vi "DP-Plot DPGram.vi"(0 "DPGram":dbl[][](array[numeric]), 1 "Plot refnum":refnum<vi>, 7 "F2":dbl[](array[numeric]), 11 "error in":errorcluster, 12 "criteria (dB)":dbl[](array[numeric])) -> (4 "DPGram thru":dbl[][](array[numeric]), 8 "F2 out":dbl[](array[numeric]), 15 "error out":errorcluster)   [LabVIEW 2020]
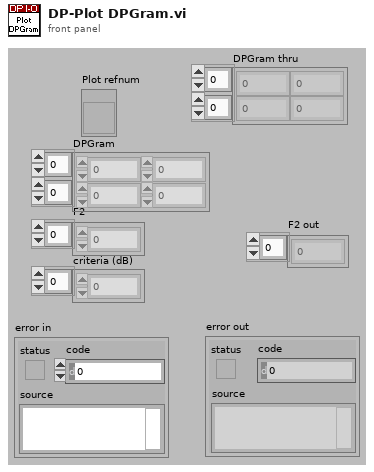
[diagram p1: front panel]
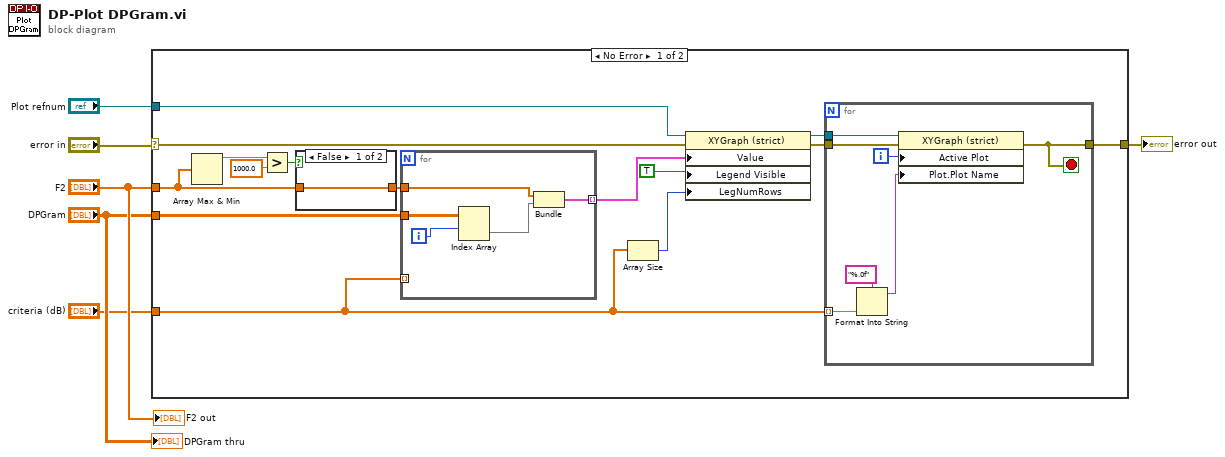
[diagram p0: block diagram]
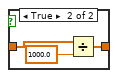
[diagram p2: hidden frame]
diagram:
  n1 = case shown="No Error" "error in" {
    selector: "error in" -> [w14 w38]
    tunnel: "DPGram" -> [w21 _]
    tunnel: "F2" -> [w10 _]
    tunnel: "Plot refnum" -> [w19 _]
    tunnel: "criteria (dB)" -> [w16 _]
    tunnel: [w12 w38] -> w1
    frame No Error {
      n2 = Array Max & Min(array=w10) -> (max value=w9:dbl)  [unwired: 3 out]
      n3 = Greater?(x=w9, y=1000.0) -> (0:w7:bool)
      n4 = case shown="False" w7 {
        tunnel: [w22 w25] -> w18
        tunnel: w10 -> [w22 w23]
        frame False {
        }
        frame True {
          n5 = Divide(x=w23, y=1000.0) -> (x/y=w25:dbl[])
        }
      }
      n6 = for {
        tunnel: w16 -> [_] mode=indexing
        tunnel: w21 -> [w37]
        tunnel: w18 -> [w36]
        tunnel: [w34] -> w20 mode=indexing
        i -> [w33]
        n7 = Index Array(array=w37, index (row)=w33) -> (element=w35:dbl[])  [unwired: 1 in]
        n8 = Bundle("F2"=w36, "DPGram"=w35) -> (w34:cluster{"F2":dbl[], "DPGram":dbl[]})  [unwired: 1 in]
      }
      n9 = Array Size(array=w16) -> (size(s)=w15:i32)
      n10 = property class="XYGraph (strict)"(reference=w19, error in=w14, "Value"=w20, "Legend Visible"=TRUE ("Legend:Visible"), "LegNumRows"=w15) -> (reference out=w17:refnum<vi>, error out=w13:errorcluster)
      n11 = for {
        tunnel: w16 -> [w30] mode=indexing
        tunnel: w17 -> [w32]
        tunnel: w13 -> [w27]
        tunnel: [w26] -> w12
        i -> [w31]
        stop <- w26 stop-if-true
        n12 = Format Into String(format string="%.0f", w30) -> (resulting string=w28:string)  [unwired: 2 in, 1 out]
        n13 = property class="XYGraph (strict)"(reference=w32, error in=w27, "Active Plot"=w31, "Plot.Plot Name"=w28) -> (error out=w26:errorcluster)  [unwired: 1 out]
      }
    }
    frame Error {
    }
  }
  "error out" <- w1
  "F2 out" <- "F2"
  "DPGram thru" <- "DPGram"
